vi "Connect.vi"(7 "Type":enum16{"Server", "Client"}(ring), 8 "error in":errorcluster, 10 "Port":u16, 11 "IP":string) -> (0 "error out":errorcluster)   [LabVIEW 2014, in "TCP.lvlib"]
uses:
  TCP.lvlib
  support/Message Queue/Message Queue.lvlib
  Support/Message Queue/Enqueue Message (Single).vi
  TypeDefs/TCP Data.ctl
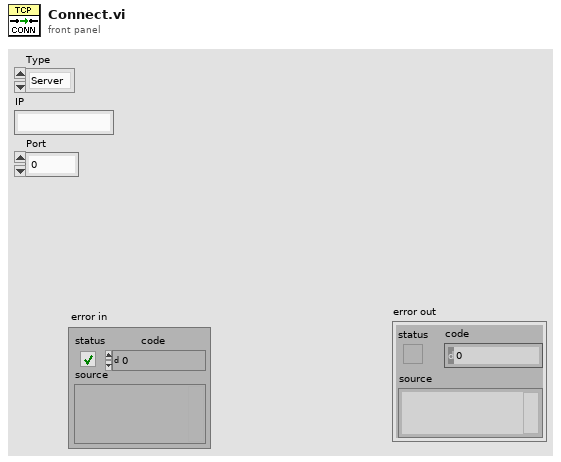
[diagram p1: front panel]
types:
  T1 = typedef "TCP.lvlib/TCP Data.ctl" = cluster{"Type":enum16{"Server", "Client"}, "IP":string, "Port":u16, "connection ID":refnum<k5>, "Connected?":bool, "Data":string}
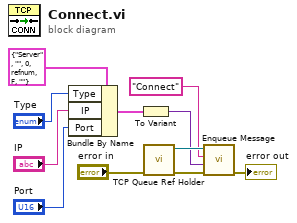
[diagram p0: block diagram]
diagram:
  n1 = Bundle By Name(cluster=T1 {"Type"=enum."Server", "IP"="", "Port"=0, "connection ID"=refnum, "Connected?"=FALSE, "Data"=""} ("TCP Data"), "Type"="Type", "IP"="IP", "Port"="Port") -> (w2:T1)
  n2 = To Variant(anything=w2) -> (Variant=w1:variant)
  n3 = call "TCP Queue Ref Holder.vi"("error in"="error in") -> ("error out"=w10:errorcluster, "Input Message Queue"=w8:refnum<queue>)  [unwired: 9 in]
  n4 = call-poly "Enqueue Message.vi"("error in (no error)"=w10, "Message Data"=w1, "Message"="Connect", "Message Queue"=w8) -> ("error out"=→"error out":errorcluster)  [unwired: 6 in, 1 out]
